vi "k_calc.vi"(2 "Cell Temp":dbl, 3 "Cell Temp Correction Formula":string="8.617384E-5*(x+273.15)") -> (0 "Corrected Cell Temp":dbl format="%.2f", 1 "k":dbl)   [LabVIEW 2010]
uses:
  <vilib>/gmath/NI_Gmath.lvlib
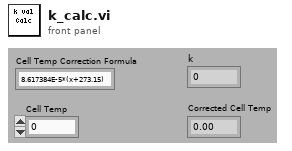
[diagram p1: front panel]
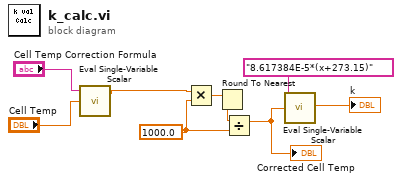
[diagram p0: block diagram]
diagram:
  w6 = 1000.0 ("y")
  n1 = call <vilib>:"Eval Single-Variable Scalar.vi"("x value"="Cell Temp", "formula"="Cell Temp Correction Formula") -> ("y value"=w2:dbl)  [unwired: 1 in, 1 out]
  n2 = Multiply(x=w2, y=w6) -> (x*y=w7:dbl)
  n3 = Round To Nearest(number=w7) -> ()  [unwired: 1 out]
  n4 = Divide(x=w7, y=w6) -> (x/y=w5:dbl)
  "Corrected Cell Temp" <- w5
  n5 = call <vilib>:"Eval Single-Variable Scalar.vi"("x value"=w5, "formula"="8.617384E-5*(x+273.15)") -> ("y value"=→"k":dbl)  [unwired: 1 in, 1 out]
